vi "dll_test.vi"() -> ()   [LabVIEW 2014]
uses:
  dll/DaliBusAccess.dll
panel:
  out "error out":errorcluster
  in  "error in (no error)":errorcluster
  out "Array":string[](array[string])
  out "DLL version":string
  out "Bus version":string
  out "return type":i32
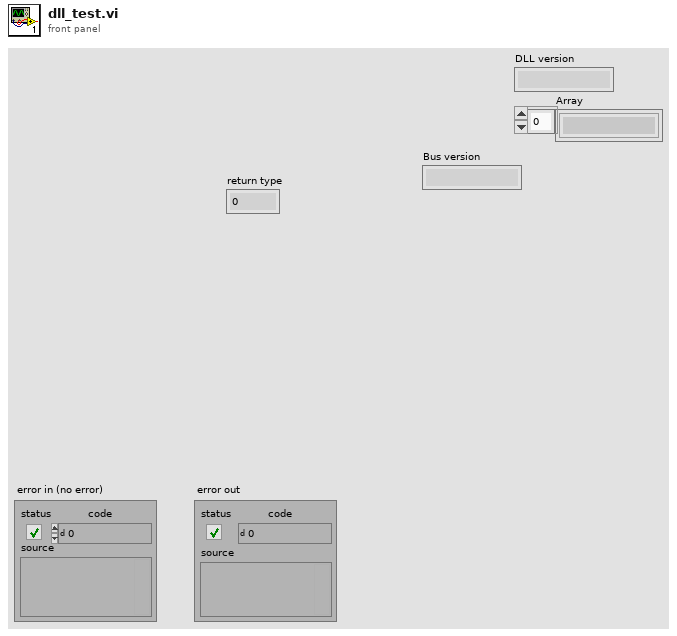
[diagram p1: front panel]
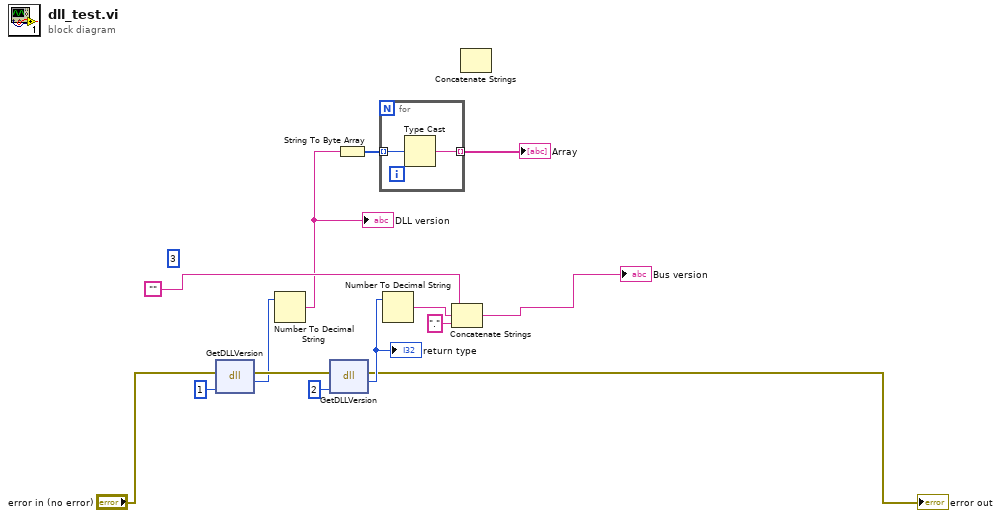
[diagram p0: block diagram]
diagram:
  (unwired) 3
  n1 = dll-call lib="C:/LTS/app-tde-luminaires/SourceCode/Instruments/Driver_interaction/Dali_usb/Vendor/dll/DaliBusAccess.dll" fn="GetDLLVersion"(error in="error in (no error)", "iIndex"=1) -> (error out=w7:errorcluster, "return type"=w6:i32)  [unwired: 3 in, 1 out]
  n2 = Number To Decimal String(number=w6) -> (decimal integer string=w5:string)  [unwired: 1 in]
  "DLL version" <- w5
  n3 = dll-call lib="C:/LTS/app-tde-luminaires/SourceCode/Instruments/Driver_interaction/Dali_usb/Vendor/dll/DaliBusAccess.dll" fn="GetDLLVersion"(error in=w7, "iIndex"=2) -> (error out=→"error out":errorcluster, "return type"=w12:i32)  [unwired: 3 in, 1 out]
  "return type" <- w12
  n4 = String To Byte Array(string=w5) -> (unsigned byte array=w4:u8[])
  n5 = for {
    tunnel: w4 -> [w16] mode=indexing
    tunnel: [w15] -> w3 mode=indexing
    n6 = Type Cast(x=w16) -> (*(type *) &x=w15:string)  [unwired: 1 in]
  }
  "Array" <- w3
  n7 = Number To Decimal String(number=w12) -> (decimal integer string=w10:string)  [unwired: 1 in]
  n8 = Concatenate Strings("", w10, "." ("string")) -> (→"Bus version":string)
  n9 = Concatenate Strings() -> ()  [unwired: 3 in, 1 out]
